vi "Draw.vi"(8 "error in (no error)":errorcluster, 9 "disable contained items?":bool, 10 "IB_Tree":refnum<class "IB_Tree.lvclass">, 11 "IB_TreeItem in":refnum<class "IB_Tree_Item_Proj_Contained_File.lvclass">) -> (0 "error out":errorcluster, 3 "IB_TreeItem out":refnum<class "IB_Tree_Item_Proj_Contained_File.lvclass">)   [LabVIEW 2020, in "IB_Tree_Item_Proj_Contained_File.lvclass"]
uses:
  <vilib>/AppBuilder/IB_Classes/Tree_Item_Proj_Contained_File/IB_Tree_Item_Proj_Contained_File.lvclass
  <vilib>/AppBuilder/IB_Classes/Tree_Item_Proj_Contained_File/IB_Tree_Item_Proj_Contained_File.lvclass/IB_Tree_Item_Proj_Contained_File.ctl
  <vilib>/AppBuilder/IB_Classes/Tree_Item_Virtual_Folder/IB_Tree_Item_Virtual_Folder.lvclass
  <vilib>/AppBuilder/IB_Classes/Tree_Item_Proj_File/IB_Tree_Item_Proj_File.lvclass
  <vilib>/AppBuilder/IB_Classes/Tree/IB_Tree.lvclass
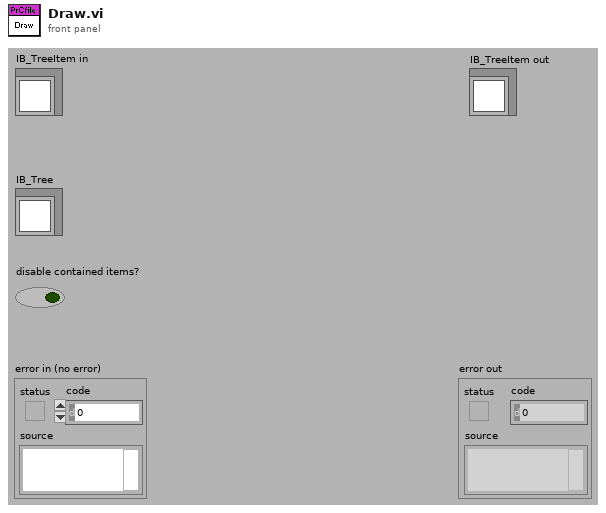
[diagram p1: front panel]
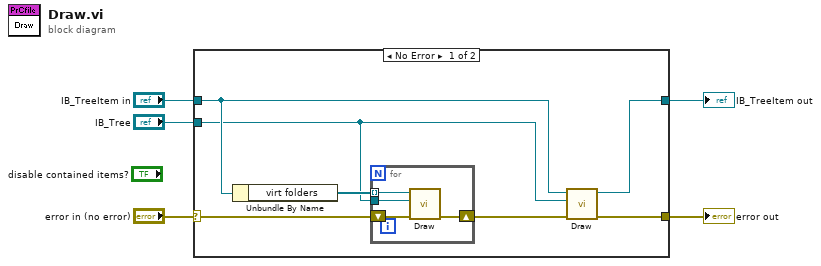
[diagram p0: block diagram]
diagram:
  n1 = case shown="No Error" "error in (no error)" {
    selector: "error in (no error)" -> [w9 w18]
    tunnel: [w12 w18] -> w5
    tunnel: [w11 w17] -> w4
    tunnel: "IB_Tree" -> [w6 _]
    tunnel: "IB_TreeItem in" -> [w10 w17]
    frame No Error {
      n2 = Unbundle By Name(w10) -> ("virt folders"=w7:refnum<class "IB_Tree_Item_Virtual_Folder.lvclass">[])
      n3 = for {
        shift-right: [w15] -> w8
        shift-left: w9 -> [w16]
        tunnel: w7 -> [w14] mode=indexing
        tunnel: w6 -> [w13]
        n4 = call-dynamic "Draw.vi"("error in (no error)"=w16, "IB_Tree"=w13, "IB_TreeItem in"=w14) -> ("error out"=w15:errorcluster)  [unwired: 1 in, 7 out]
      }
      n5 = call-parent "Draw.vi"("error in (no error)"=w8, "IB_Tree"=w6, "IB_TreeItem in"=w10) -> ("error out"=w12:errorcluster, "IB_TreeItem out"=w11:refnum<class "IB_Tree_Item_Proj_Contained_File.lvclass">)  [unwired: 1 in, 6 out]
    }
    frame Error {
    }
  }
  "error out" <- w5
  "IB_TreeItem out" <- w4
